vi "Get All Routing Channel Ref IDs.vi"(8 "error in (no error)":errorcluster, 11 "Routing Channels Ref in":T1 format="%.0x") -> (0 "error out":errorcluster, 2 "Channel Refs":T1[](array[typedef]) format="%.0x", 3 "Routing Channels Ref out":T1 format="%.0x")   [LabVIEW 2017, in "Routing and Faulting Scripting.lvlib"]
uses:
  Routing and Faulting Scripting.lvlib
  <vilib>/NI Veristand/Custom Device API/Custom Device Item Ref.ctl
  <vilib>/NI Veristand/Custom Device Tools/Custom Device Utility Library/Custom Device Utility Library.lvlib
  <vilib>/NI VeriStand/Custom Device API/Custom Device API.lvlib
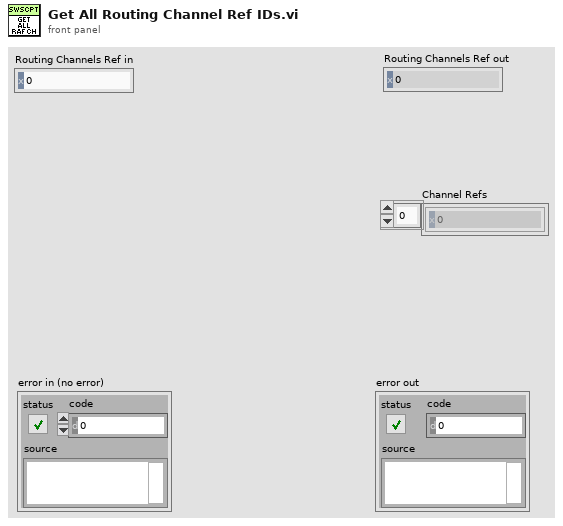
[diagram p1: front panel]
types:
  T1 = typedef "Custom Device API.lvlib/Custom Device Item Ref.ctl" = u64
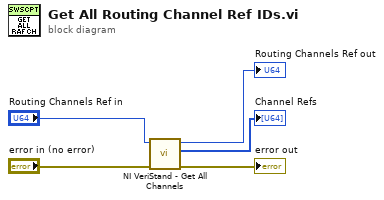
[diagram p0: block diagram]
diagram:
  n1 = call <vilib>:"NI VeriStand - Get All Channels.vi"("error in"="error in (no error)", "Section Ref in"="Routing Channels Ref in") -> ("error out"=→"error out":errorcluster, "Channel Refs"=→"Channel Refs":T1[], "Section Ref out"=→"Routing Channels Ref out":T1)  [unwired: 6 in, 1 out]
